vi "unregisterServiceReply.vi"(2 "Service":T1, 3 "error in":errorcluster) -> (0 "XML":string)   [LabVIEW 2013, in "ROS_Master.lvclass"]
uses:
  <userlib>/ROSforLV/ROS/Code/SubVIs/ROS_Master/ROS_Master.lvclass
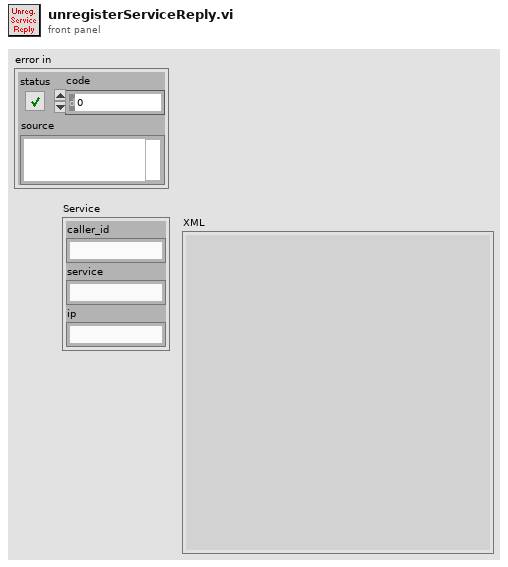
[diagram p1: front panel]
types:
  T1 = cluster{"caller_id":string, "service":string, "ip":string}
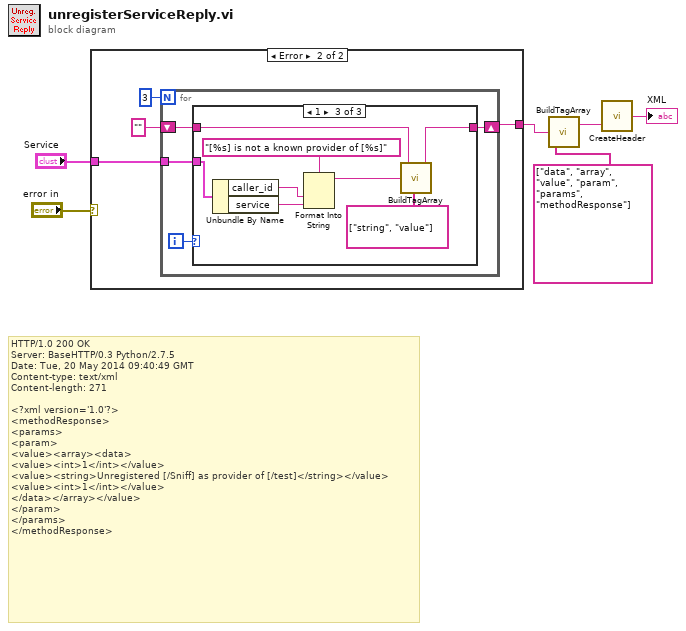
[diagram p0: block diagram]
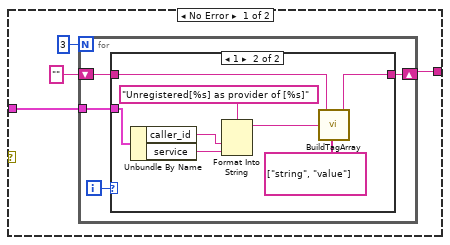
[diagram p2: hidden frame]
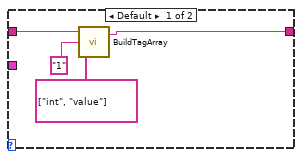
[diagram p3: hidden frame]
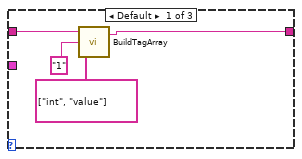
[diagram p4: hidden frame]
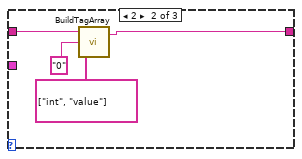
[diagram p5: hidden frame]
diagram:
  # "HTTP/1.0 200 OK\nServer: BaseHTTP/0.3 Python/2.7.5\nDate: Tue, 20 May 2014 09:40:49 GMT\nContent-type: text/xml\nContent-length: 271\n\n<?xml version='1.0'?>\n<methodResponse>\n<params>\n<param>\n<value><array><data>\n<value><int>1</int></value>\n<value><string>Unregistered [/Sniff] as provider of [/test]</string></value>\n<value><int>1</int></value>\n</data></array></value>\n</param>\n</params>\n</methodResponse>"
  n1 = case shown="Error" "error in" {
    tunnel: "Service" -> [w8 w28]
    tunnel: [w7 w27] -> w3
    frame No Error {
      n2 = for {
        N: 3 -> [_]
        shift-right: [w11] -> w7
        shift-left: "" ("caller_id") -> [w13]
        tunnel: w8 -> [w12]
        i -> [w14]
        n3 = case shown="1" w14 {
          tunnel: w13 -> [w16 w20]
          tunnel: w12 -> [_ w25]
          tunnel: [w15 w19] -> w11
          frame Default {
            n4 = call <userlib>:"BuildTagArray.vi"("tags"=string[] ["int", "value"], "value"="1", "string in"=w16) -> ("string out"=w15:string)  [unwired: 1 in]
          }
          frame 1 {
            n5 = Unbundle By Name(w25) -> ("caller_id"=w23:string, "service"=w22:string)
            n6 = Format Into String(format string="Unregistered[%s] as provider of [%s]", w23, w22) -> (resulting string=w21:string)  [unwired: 2 in, 1 out]
            n7 = call <userlib>:"BuildTagArray.vi"("tags"=string[] ["string", "value"], "value"=w21, "string in"=w20) -> ("string out"=w19:string)  [unwired: 1 in]
          }
        }
      }
    }
    frame Error {
      n8 = for {
        N: 3 -> [_]
        shift-right: [w31] -> w27
        shift-left: "" ("caller_id") -> [w33]
        tunnel: w28 -> [w32]
        i -> [w34]
        n9 = case shown="1" w34 {
          tunnel: w33 -> [w36 w40 w44]
          tunnel: w32 -> [_ _ w49]
          tunnel: [w35 w39 w43] -> w31
          frame Default {
            n10 = call <userlib>:"BuildTagArray.vi"("tags"=string[] ["int", "value"], "value"="1", "string in"=w36) -> ("string out"=w35:string)  [unwired: 1 in]
          }
          frame 2 {
            n11 = call <userlib>:"BuildTagArray.vi"("tags"=string[] ["int", "value"], "value"="0", "string in"=w40) -> ("string out"=w39:string)  [unwired: 1 in]
          }
          frame 1 {
            n12 = Unbundle By Name(w49) -> ("caller_id"=w47:string, "service"=w46:string)
            n13 = Format Into String(format string="[%s] is not a known provider of [%s]", w47, w46) -> (resulting string=w45:string)  [unwired: 2 in, 1 out]
            n14 = call <userlib>:"BuildTagArray.vi"("tags"=string[] ["string", "value"], "value"=w45, "string in"=w44) -> ("string out"=w43:string)  [unwired: 1 in]
          }
        }
      }
    }
  }
  n15 = call <userlib>:"BuildTagArray.vi"("tags"=string[] ["data", "array", "value", "param", "params", "methodResponse"], "value"=w3) -> ("string out"=w2:string)  [unwired: 2 in]
  n16 = call <userlib>:"CreateHeader.vi"("Content"=w2) -> ("XML"=→"XML":string)  [unwired: 1 in]
